vi "collectInfo.vi"(6 "Value":string, 8 "error in (no error)":errorcluster, 9 "Dt":dbl, 10 "Time":dbl, 11 "playFileAction in":refnum<class "playFileAction.lvclass">) -> (0 "error out":errorcluster, 3 "playFileAction out":refnum<class "playFileAction.lvclass">)   [LabVIEW 2011, in "Views.lvlib" / "ScriptEditor.lvlib" / "playFileAction.lvclass"]
uses:
  playFileAction.lvclass
  Tools/Scripting/ScriptingEvent/ScriptEvents/PlayFile/PlayFile.lvclass
  playFileAction.lvclass/playFileAction.ctl
  Tools/Scripting/ScriptingEvent/ScriptEvent.lvclass
  ActionPanel.lvclass
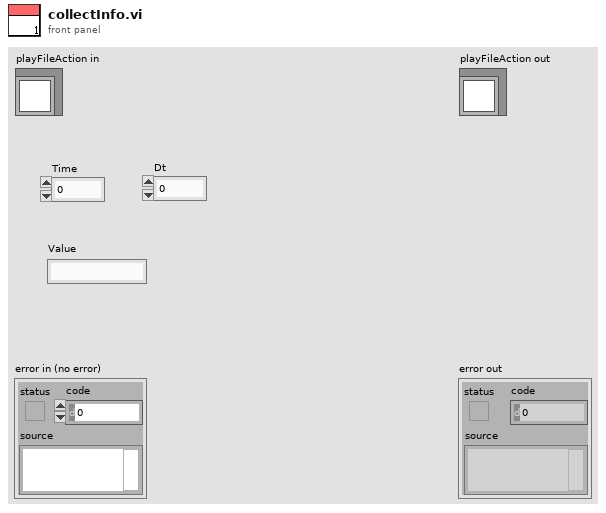
[diagram p1: front panel]
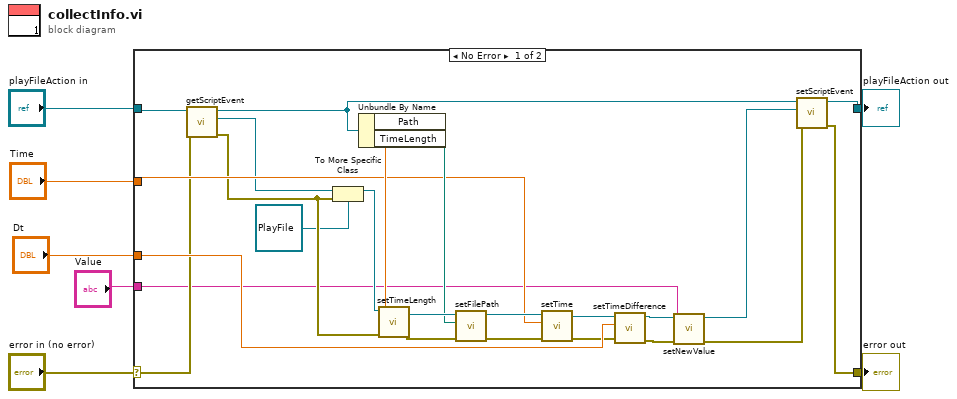
[diagram p0: block diagram]
diagram:
  n1 = case shown="No Error" "error in (no error)" {
    selector: "error in (no error)" -> [w20 w33]
    tunnel: [w14 w33] -> w6
    tunnel: [w13 w32] -> w4
    tunnel: "playFileAction in" -> [w21 w32]
    tunnel: "Time" -> [w25 _]
    tunnel: "Dt" -> [w26 _]
    tunnel: "Value" -> [w8 _]
    frame No Error {
      n2 = call "getScriptEvent.vi"("error in (no error)"=w20, "ActionPanel.lvclass in"=w21) -> ("error out"=w17:errorcluster, "ScriptEvent.lvclass"=w19:refnum<class "ScriptEvent.lvclass">, "ActionPanel.lvclass out"=w15:refnum<class "playFileAction.lvclass">)  [unwired: 7 in]
      n3 = To More Specific Class(target class=refnum<class "PlayFile.lvclass"> refnum ("PlayFile out"), reference=w19, error in=w17) -> (specific class reference=w18:refnum<class "PlayFile.lvclass">)  [unwired: 1 out]
      n4 = Unbundle By Name(w15) -> ("Path"=w29:path, "TimeLength"=w30:dbl)
      n5 = call "setTimeLength.vi"("error in (no error)"=w17, "timeLength"=w30, "PlayFile in"=w18) -> ("error out"=w22:errorcluster, "PlayFile out"=w31:refnum<class "PlayFile.lvclass">)  [unwired: 7 in]
      n6 = call "setFilePath.vi"("error in (no error)"=w22, "filePath"=w29, "PlayFile in"=w31) -> ("error out"=w24:errorcluster, "PlayFile out"=w28:refnum<class "PlayFile.lvclass">)  [unwired: 7 in]
      n7 = call "setTime.vi"("error in (no error)"=w24, "time"=w25, "ScriptEvent.lvclass in"=w28) -> ("error out"=w23:errorcluster, "ScriptEvent.lvclass out"=w27:refnum<class "PlayFile.lvclass">)  [unwired: 7 in]
      n8 = call "setTimeDifference.vi"("error in (no error)"=w23, "time difference"=w26, "ScriptEvent.lvclass in"=w27) -> ("error out"=w11:errorcluster, "ScriptEvent.lvclass out"=w12:refnum<class "PlayFile.lvclass">)  [unwired: 7 in]
      n9 = call "setNewValue.vi"("error in (no error)"=w11, "newValue"=w8, "ScriptEvent.lvclass in"=w12) -> ("error out"=w9:errorcluster, "ScriptEvent.lvclass out"=w10:refnum<class "PlayFile.lvclass">)  [unwired: 7 in]
      n10 = call "setScriptEvent.vi"("error in (no error)"=w9, "ScriptEvent.lvclass"=w10, "ActionPanel.lvclass in"=w15) -> ("error out"=w14:errorcluster, "ActionPanel.lvclass out"=w13:refnum<class "playFileAction.lvclass">)  [unwired: 7 in]
    }
    frame Error {
    }
  }
  "error out" <- w6
  "playFileAction out" <- w4
